vi "Analys UP.vi"(8 "error in":errorcluster, 11 "data":T1) -> (0 "error out":errorcluster, 2 "output cluster":cluster{"Array":dbl[], "Array":dbl[]})   [LabVIEW 2019]
uses:
  UPLINK/Analys Argument--cluster.ctl
  TypeDef/Analys data.ctl
  TypeDef/Analys type.ctl
  TypeDef/Sett data.ctl
  TypeDef/ISO.ctl
  TypeDef/Noise.ctl
  TypeDef/Link.ctl
  Class/ISO 14443 A UP.lvclass
  Class/ISO 14443 B UP.lvclass
  Class/Felica UP.lvclass
  Class/ISO 15693 UP.lvclass
  UPLINK/UPLINK.lvlib
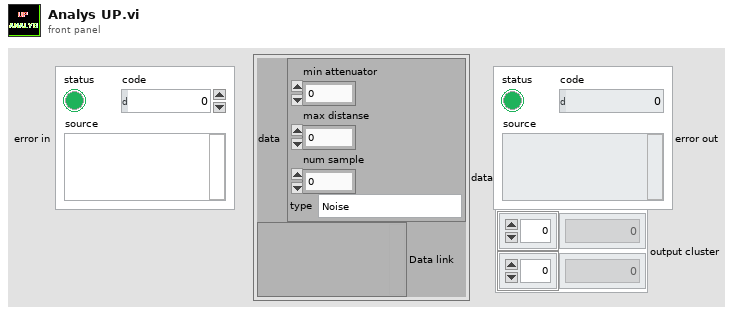
[diagram p1: front panel]
types:
  T1 = typedef "UPLINK.lvlib/Analys Argument--cluster.ctl" = cluster{"data":T2, "Data link":variant}
  T2 = typedef "Analys data.ctl" = cluster{"min attenuator":dbl, "max distanse":dbl, "num sample":dbl, "type":T3}
  T3 = typedef "Analys type.ctl" = enum16{"Noise", "Distance"}
  T4 = typedef "Sett data.ctl" = cluster{"Filter":i32, "Gain":dbl, "Bit rate":dbl, "ISO/IEC w ":T5, "BI":cluster{"R":dbl, "C":dbl, "L":dbl}, "BM":cluster{"R":dbl, "C":dbl, "L":dbl}, "M":cluster{"Метка":i64, "Считыветель":i64}, "Type noise":T6, "Link":T7, "Noise attenuator":dbl, "Signal gain":dbl, "Distance":dbl}
  T5 = typedef "ISO.ctl" = enum16{"14443 Type A", "14443 Type B", "Felica", "15693"}
  T6 = typedef "Noise.ctl" = enum16{"Гауссовский шум", "Белый шум"}
  T7 = typedef "Link.ctl" = enum16{"UPLINK", "DOWNLINK"}
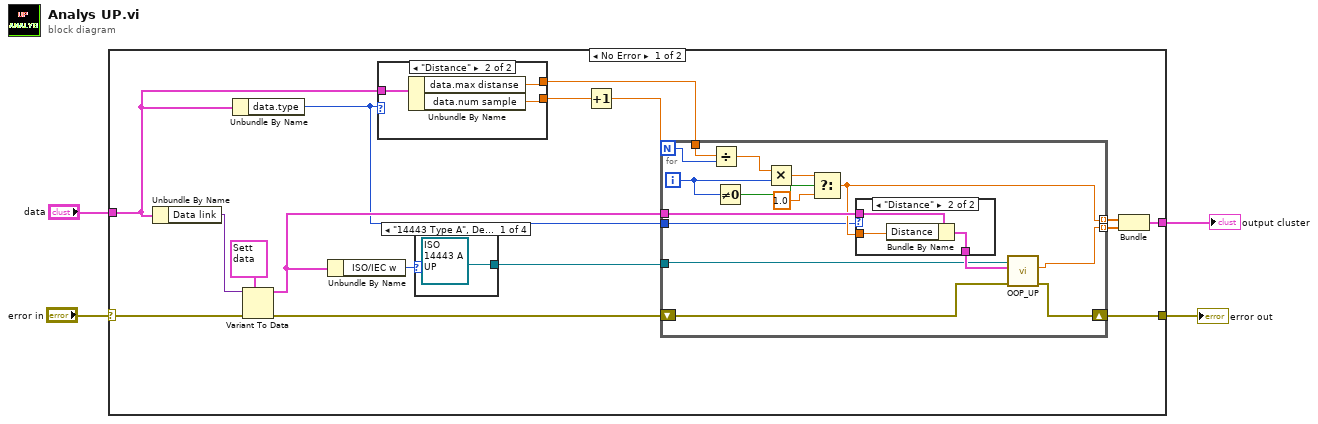
[diagram p0: block diagram]
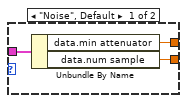
[diagram p2: hidden frame]
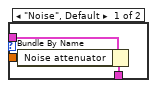
[diagram p3: hidden frame]
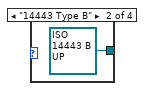
[diagram p4: hidden frame]
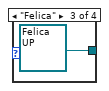
[diagram p5: hidden frame]
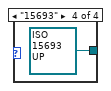
[diagram p6: hidden frame]
diagram:
  n1 = case shown="No Error" "error in" {
    selector: "error in" -> [w17 w52]
    tunnel: [w8 w52] -> w4
    tunnel: "data" -> [w7 _]
    tunnel: [w16 _] -> w1
    frame No Error {
      n2 = Unbundle By Name(w7) -> ("Data link"=w19:variant)
      n3 = Unbundle By Name(w7) -> ("data.type"=w6:T3)
      n4 = Variant To Data(error in=w17, type=T4 {"Filter"=0, "Gain"=0.0, "Bit rate"=0.0, "ISO/IEC w "=enum."14443 Type A", "BI"={"R"=0.0, "C"=0.0, "L"=0.0}, "BM"={"R"=0.0, "C"=0.0, "L"=0.0}, "M"={"Метка"=4, "Считыветель"=4}, "Type noise"=enum."Гауссовский шум", "Link"=enum."UPLINK", "Noise attenuator"=0.0, "Signal gain"=1.0, "Distance"=0.0} ("Sett data"), Variant=w19) -> (data=w13:T4, error out=w15:errorcluster)
      n5 = Unbundle By Name(w13) -> ("ISO/IEC w"=w20:T5)
      n6 = case shown="\"Distance\"" w6 {
        tunnel: [w23 w24] -> w12
        tunnel: [w22 w25] -> w11
        tunnel: w7 -> [w21 w26]
        frame "Noise", Default {
          n7 = Unbundle By Name(w21) -> ("data.min attenuator"=w22:dbl, "data.num sample"=w23:dbl)
        }
        frame "Distance" {
          n8 = Unbundle By Name(w26) -> ("data.max distanse"=w25:dbl, "data.num sample"=w24:dbl)
        }
      }
      n9 = case shown="\"14443 Type A\", Default" w20 {
        tunnel: [refnum<class "ISO 14443 A UP.lvclass"> refnum ("ISO 14443 A UP.lvclass") refnum<class "ISO 14443 B UP.lvclass"> refnum ("ISO 14443 B UP.lvclass") refnum<class "Felica UP.lvclass"> refnum ("Felica UP.lvclass") refnum<class "ISO 15693 UP.lvclass"> refnum ("ISO 15693 UP.lvclass")] -> w14
        frame "14443 Type A", Default {
        }
        frame "14443 Type B" {
        }
        frame "Felica" {
        }
        frame "15693" {
        }
      }
      n10 = Increment(x=w12) -> (x+1=w5:dbl)
      n11 = for {
        N: w5 -> [w41]
        shift-right: [w31] -> w8
        shift-left: w15 -> [w32]
        tunnel: w14 -> [w29]
        tunnel: w13 -> [w39]
        tunnel: [w33] -> w10 mode=indexing
        tunnel: [w28] -> w9 mode=indexing
        tunnel: w11 -> [w38]
        tunnel: w6 -> [w27]
        i -> [w36]
        n12 = Divide(x=w38, y=w41) -> (x/y=w40:dbl)
        n13 = Not Equal To 0?(x=w36) -> (x != 0?=w37:bool)
        n14 = Multiply(x=w40, y=w36) -> (x*y=w34:dbl)
        n15 = Select(t=w34, s=w37, f=1.0) -> (s? t:f=w33:dbl)
        n16 = case shown="\"Distance\"" w27 {
          tunnel: w39 -> [w44 w47]
          tunnel: w33 -> [w43 w45]
          tunnel: [w42 w46] -> w30
          frame "Noise", Default {
            n17 = Bundle By Name(cluster=w44, "Noise attenuator"=w43) -> (w42:T4)
          }
          frame "Distance" {
            n18 = Bundle By Name(cluster=w47, "Distance"=w45) -> (w46:T4)
          }
        }
        n19 = call "OOP_UP.vi"("error in (no error)"=w32, "Sett data"=w30, "RFID system in"=w29) -> ("error out"=w31:errorcluster, "Error on  byte"=w28:dbl)  [unwired: 6 in, 1 out]
      }
      n20 = Bundle(w10, w9) -> (w16:cluster{dbl[], dbl[]})  [unwired: 1 in]
    }
    frame Error {
    }
  }
  "error out" <- w4
  "output cluster" <- w1
